vi "DashboardPush.vi"(5 "Joystick 0 Ref":T1, 7 "Joystick 1 Ref":T1) -> ()   [LabVIEW 2018]
uses:
  <vilib>/Rock Robotics/WPI/Joystick/WPI_JoystickDevRef.ctl
  <vilib>/Rock Robotics/WPI/Joystick/WPI_JoystickDeviceEnum.ctl
  1cd4df9d-07b4-47b1-9361-2cbb9b342794.vi
  3ad63815-9e92-4927-9537-e4f1665bbc86.vi
  3818bb57-508c-4caa-99a3-3627e757767c.vi
  6295dfb8-7bb5-4d21-8815-7d68ced149fe.vi
  69aab131-d86d-4f55-ad43-4766d5f58e80.vi
  c3e94fa6-8c65-408c-b4b8-dd7b71f991a8.vi
  26d44c84-0892-4d1c-ad1a-86279a09e0cc.vi
  6918a5f6-b485-4e67-ab72-405280ef4693.vi
  11adc3a0-d4d2-454d-8758-117694ddcb4c.vi
  1a812ba0-d878-476d-99f2-b93886c55b51.vi
  4ab55bdd-9685-40f0-9085-ecc7bf01abd7.vi
  133b72f1-f6b5-40a0-849f-8c3469abb341.vi
  418ca814-9bf7-4181-a5ae-ea4e15d15a62.vi
  5b9a1c80-d2af-4722-947b-ad6779bb500a.vi
  bbae46cd-89b0-4a78-83b4-a5d1ddadd6d9.vi
  6394f793-1348-457d-85f4-7648f9013d39.vi
  47d326fc-03e5-451f-ae34-c9ea74063880.vi
  a9e42ba8-a108-4121-8da4-7ed463bc445a.vi
  e7382db6-2398-4bf7-9509-2739849d011a.vi
  fb3d1e40-1309-4105-9d60-3501161224b8.vi
  edb44874-fd78-454c-9bff-6d2a69ee6fec.vi
  dfb785ac-7a80-4692-ab1e-e9791fae54f3.vi
  5b13cb5e-6146-47d8-ae09-8b12801406e1.vi
  221b1552-0cc4-4389-bc13-d572fc4176ac.vi
  30f734cc-7591-4d07-939c-c5b43ee5df0c.vi
  d7311573-fb90-4913-8cda-848d1d3ce53b.vi
  7ba6df12-c395-4848-b3a1-04dcd1203c1b.vi
  6301e614-6b7f-47cf-b382-4b27c7e33111.vi
  d83519f1-9582-40c6-a23b-344b6b305b5b.vi
  6aad11fd-ae03-4511-b650-1fa0753debfc.vi
  3bc1cfba-3c18-4848-9658-0328ea52b25d.vi
  ee07aba5-9db9-42ab-a6d0-ff6a71bb383e.vi
  31b97e73-c245-4c28-83b2-b8b7bc5cac65.vi
  8687fe65-8d2d-4f02-ae89-6e8600396bf0.vi
  359c22e3-9c88-41c1-8194-a7f6db251ab3.vi
  9a35cad7-8924-4936-b892-f51ff88f3087.vi
  77a43352-c56d-4a82-a601-0e029bfbecdd.vi
  6c32de76-4603-4c98-9548-18c068db77e4.vi
  fb2c5630-2057-4e14-823f-31378c39dbf8.vi
  d6cbd67f-9b17-42bf-843e-f5ce2d93bab6.vi
  9a319e29-0bce-4b5a-a8ba-81b1ec785933.vi
  c84b3921-0e7b-4db5-8b5b-9ca439e6cec8.vi
  80ca6acc-a426-4631-8635-04e987b8dcbd.vi
  32f607b5-8f1a-4da3-a9f3-63ceddb82894.vi
  SensorReadings.vi
  RobotStates.vi
  Inputs_DriverStation.vi
  <vilib>/Rock Robotics/Network Tables/NT Write Number.vi
  <vilib>/Rock Robotics/Network Tables/NT Write Boolean.vi
  Robot Global Data.vi
  <vilib>/Rock Robotics/Network Tables/NT Write String.vi
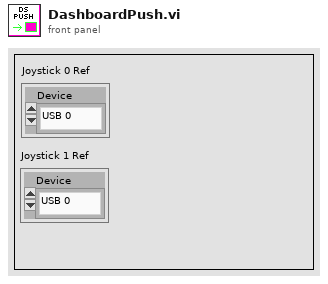
[diagram p1: front panel]
types:
  T1 = typedef "WPI_JoystickDevRef.ctl" = cluster{"Device":T2}
  T2 = typedef "WPI_JoystickDeviceEnum.ctl" = enum16{"USB 0", "USB 1", "USB 2", "USB 3", "USB 4", "USB 5"}
  T3 = cluster{"[0]":bool, "[1]":bool, "[2]":bool, "[3]":bool, "[4]":bool, "[5]":bool, "[6]":bool, "[7]":bool, "[8]":bool, "[9]":bool, "[10]":bool, "[11]":bool, "[12]":bool, "[13]":bool}
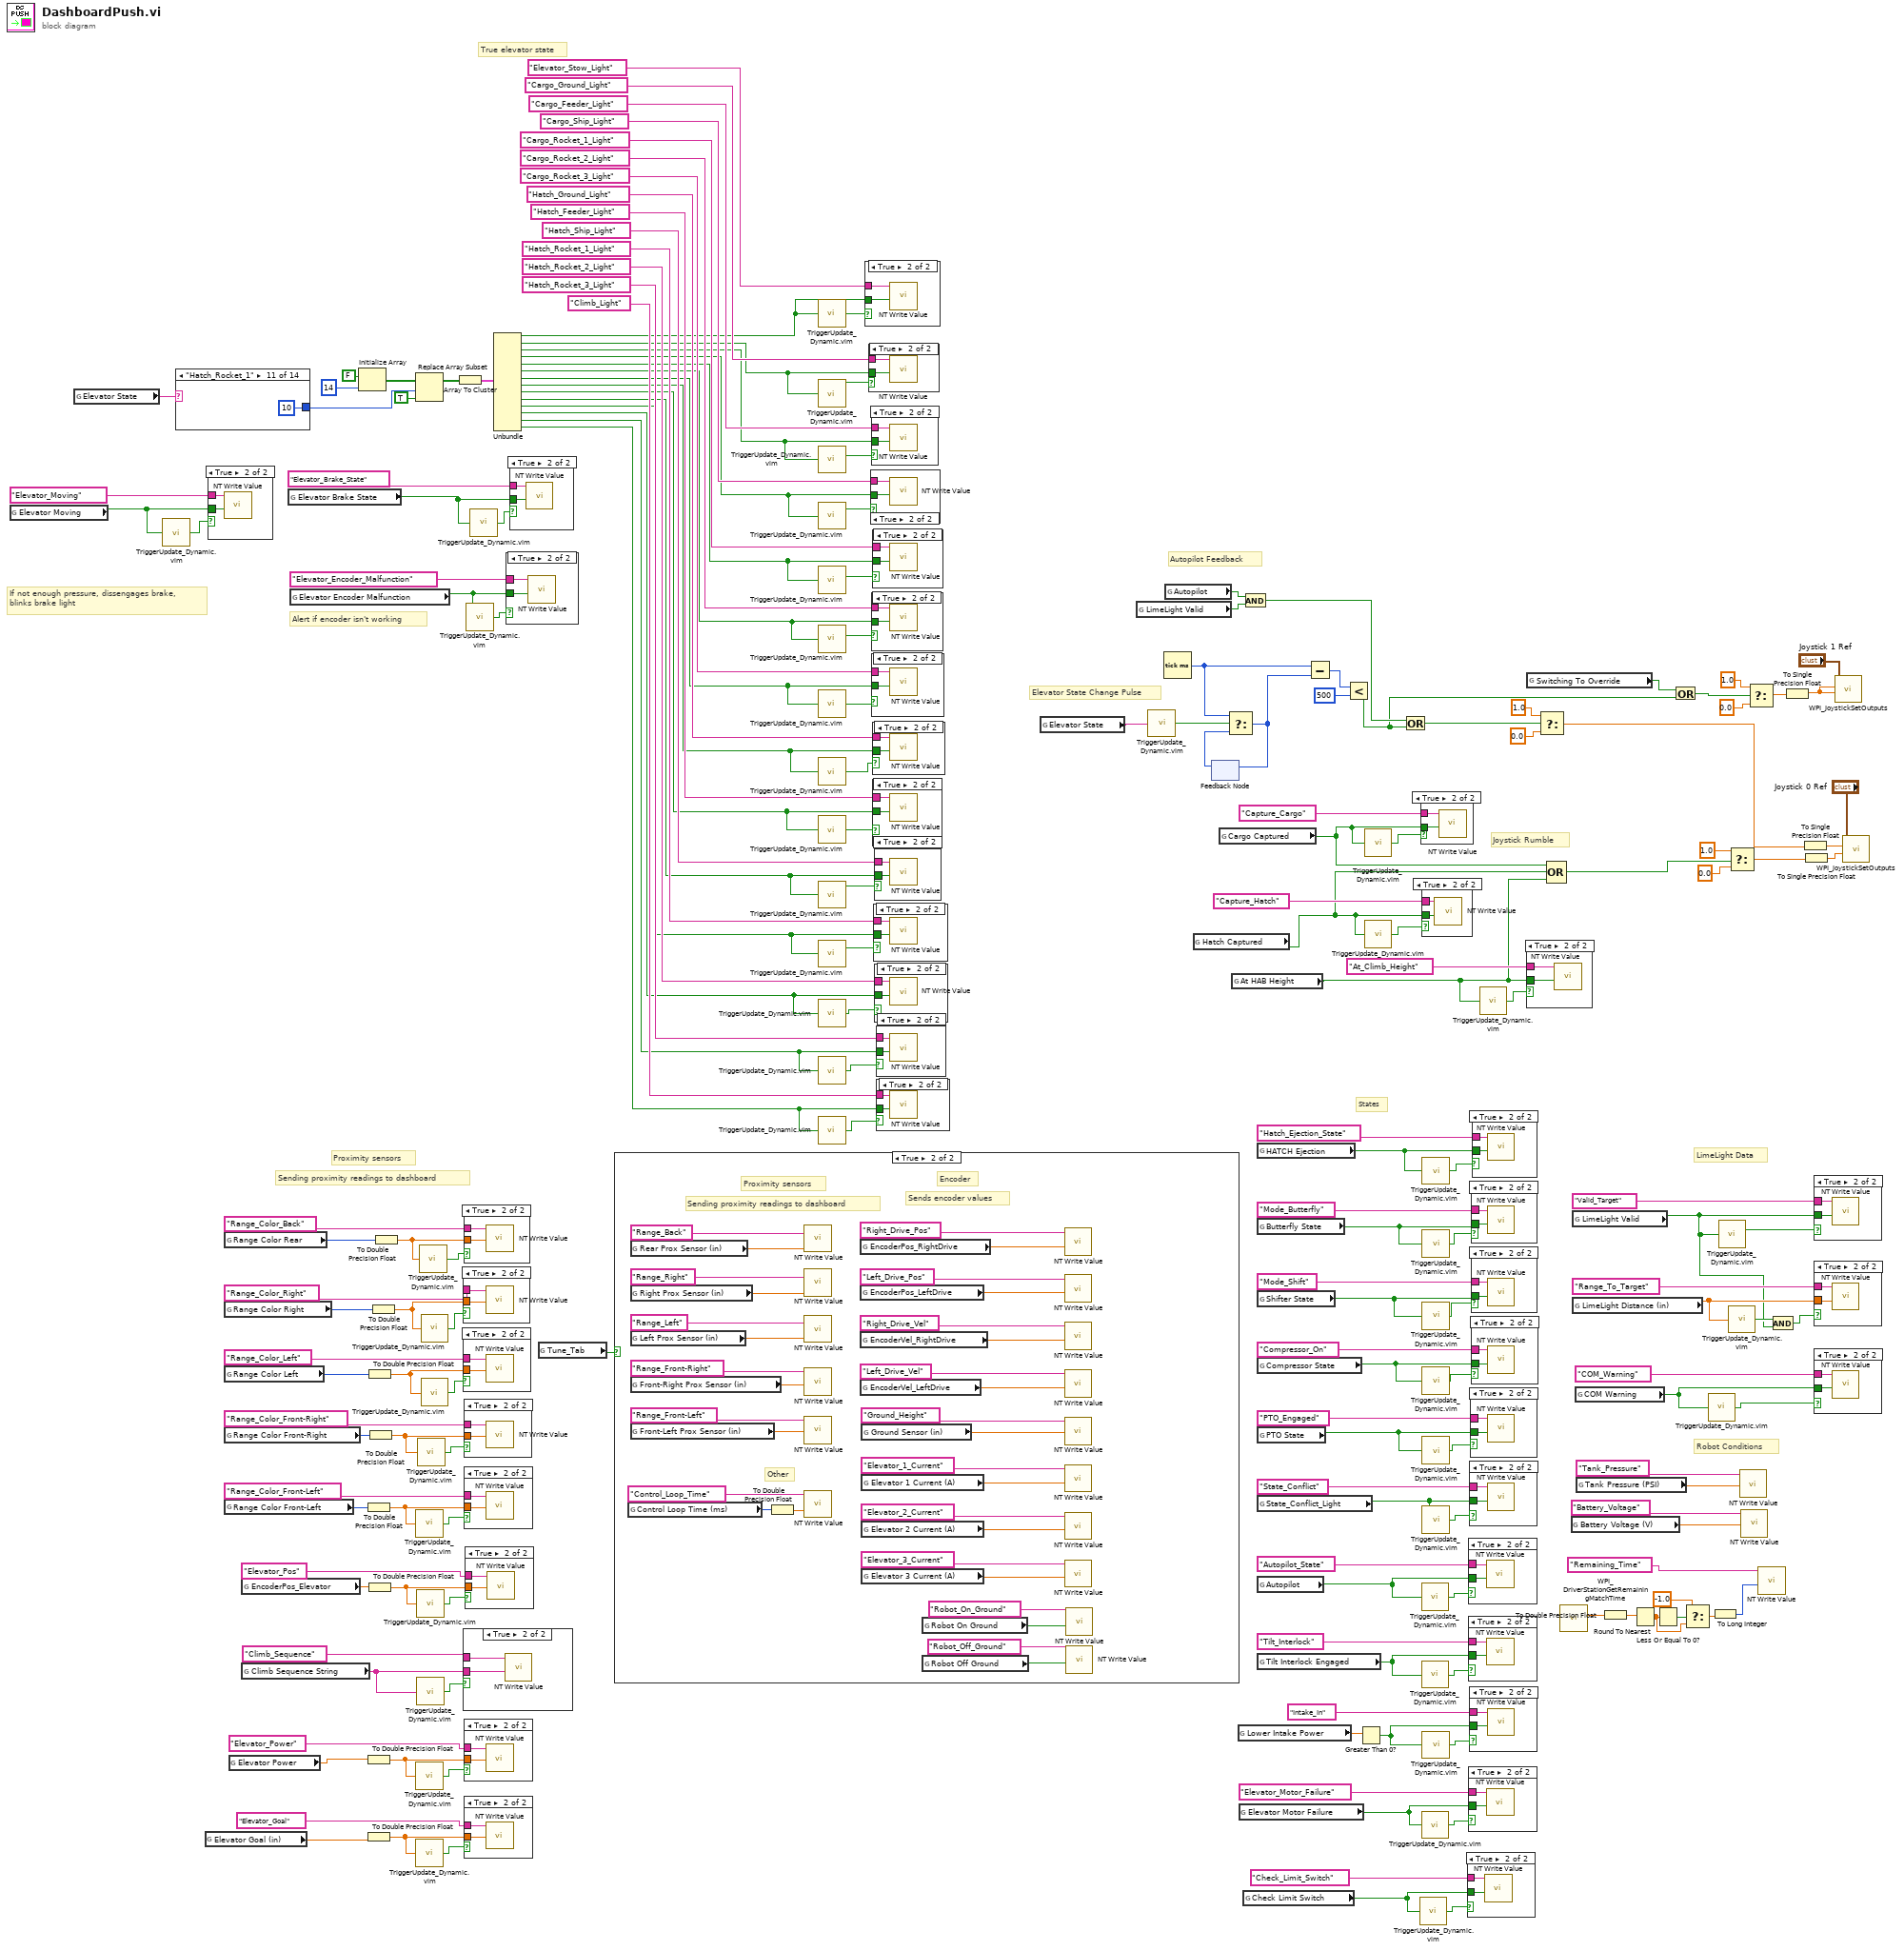
[diagram p0: block diagram]
diagram:
  # "Robot Conditions"
  # "States"
  # "Elevator State Change Pulse"
  # "LimeLight Data"
  # "Autopilot Feedback"
  # "Sending proximity readings to dashboard"
  # "Alert if encoder isn't working"
  # "If not enough pressure, dissengages brake,\nblinks brake light"
  # "Joystick Rumble"
  # "Proximity sensors"
  # "True elevator state"
  n1 = global read "RobotStates.vi" "Elevator Moving"() -> (w50:bool)
  n2 = global read "RobotStates.vi" "Elevator State"() -> (w156:string)
  n3 = call "TriggerUpdate_Dynamic.vim"("Trigger"=w50) -> ("Update"=w49:bool)
  n4 = case shown="\"Hatch_Rocket_1\"" w156 {
    tunnel: [0 1 2 3 4 5 6 7 8 9 10 11 12 13] -> w155
    frame "Elevator_Stow", Default {
    }
    frame "Cargo_Ground" {
    }
    frame "Cargo_Feeder" {
    }
    frame "Cargo_Ship" {
    }
    frame "Cargo_Rocket_1" {
    }
    frame "Cargo_Rocket_2" {
    }
    frame "Cargo_Rocket_3" {
    }
    frame "Hatch_Ground" {
    }
    frame "Hatch_Feeder" {
    }
    frame "Hatch_Ship" {
    }
    frame "Hatch_Rocket_1" {
    }
    frame "Hatch_Rocket_2" {
    }
    frame "Hatch_Rocket_3" {
    }
    frame "Climb" {
    }
  }
  n5 = global read "RobotStates.vi" "Elevator Goal (in)"() -> (w7:dbl)
  n6 = case shown="True" w49 {
    tunnel: "Elevator_Moving" ("Name") -> [_ w205]
    tunnel: w50 -> [_ w204]
    frame False {
    }
    frame True {
      n7 = call-poly <vilib>:"NT Write Value.vi"("Boolean"=w204, "Name"=w205) -> ()  [unwired: 9 in, 1 out]
    }
  }
  n8 = global read "SensorReadings.vi" "Range Color Rear"() -> (w182:u32)
  n9 = global read "SensorReadings.vi" "Range Color Right"() -> (w180:u32)
  n10 = global read "SensorReadings.vi" "Range Color Left"() -> (w178:u32)
  n11 = global read "SensorReadings.vi" "Range Color Front-Right"() -> (w176:u32)
  n12 = global read "SensorReadings.vi" "Range Color Front-Left"() -> (w151:u32)
  n13 = global read "RobotStates.vi" "Elevator Power"() -> (w11:dbl)
  n14 = global read "SensorReadings.vi" "EncoderPos_Elevator"() -> (w30:dbl)
  n15 = global read "RobotStates.vi" "Climb Sequence String"() -> (w27:string)
  n16 = global read "RobotStates.vi" "Elevator Brake State"() -> (w91:bool)
  n17 = global read "SensorReadings.vi" "Elevator Encoder Malfunction"() -> (w45:bool)
  n18 = Initialize Array(FALSE, 14 ("dimension size")) -> (w161:bool[])
  n19 = To Double Precision Float(number=w151) -> (double precision float=w95:dbl)
  n20 = To Double Precision Float(number=w11) -> (double precision float=w14:dbl)
  n21 = To Double Precision Float(number=w7) -> (double precision float=w10:dbl)
  n22 = To Double Precision Float(number=w178) -> (double precision float=w99:dbl)
  n23 = To Double Precision Float(number=w30) -> (double precision float=w33:dbl)
  n24 = To Double Precision Float(number=w176) -> (double precision float=w97:dbl)
  n25 = To Double Precision Float(number=w180) -> (double precision float=w101:dbl)
  n26 = To Double Precision Float(number=w182) -> (double precision float=w103:dbl)
  n27 = Replace Array Subset(array=w161, new element=TRUE ("new element/subarray"), index=w155) -> (w159:bool[])
  n28 = call "TriggerUpdate_Dynamic.vim"("Trigger"=w95) -> ("Update"=w94:bool)
  n29 = call "TriggerUpdate_Dynamic.vim"("Trigger"=w14) -> ("Update"=w13:bool)
  n30 = call "TriggerUpdate_Dynamic.vim"("Trigger"=w10) -> ("Update"=w9:bool)
  n31 = call "TriggerUpdate_Dynamic.vim"("Trigger"=w33) -> ("Update"=w32:bool)
  n32 = call "TriggerUpdate_Dynamic.vim"("Trigger"=w27) -> ("Update"=w29:bool)
  n33 = call "TriggerUpdate_Dynamic.vim"("Trigger"=w97) -> ("Update"=w96:bool)
  n34 = call "TriggerUpdate_Dynamic.vim"("Trigger"=w103) -> ("Update"=w102:bool)
  n35 = call "TriggerUpdate_Dynamic.vim"("Trigger"=w101) -> ("Update"=w100:bool)
  n36 = call "TriggerUpdate_Dynamic.vim"("Trigger"=w99) -> ("Update"=w98:bool)
  n37 = Array To Cluster(array=w159) -> (cluster=w158:T3)
  n38 = case shown="True" w100 {
    tunnel: "Range_Color_Right" ("refnum name") -> [_ w207]
    tunnel: w101 -> [_ w206]
    frame False {
    }
    frame True {
      n39 = call-poly <vilib>:"NT Write Value.vi"("Numeric"=w206, "Name"=w207) -> ()  [unwired: 9 in, 1 out]
    }
  }
  n40 = case shown="True" w98 {
    tunnel: "Range_Color_Left" ("refnum name") -> [_ w209]
    tunnel: w99 -> [_ w208]
    frame False {
    }
    frame True {
      n41 = call-poly <vilib>:"NT Write Value.vi"("Numeric"=w208, "Name"=w209) -> ()  [unwired: 9 in, 1 out]
    }
  }
  n42 = case shown="True" w29 {
    tunnel: "Climb_Sequence" ("Name") -> [_ w211]
    tunnel: w27 -> [_ w210]
    frame False {
    }
    frame True {
      n43 = call-poly <vilib>:"NT Write Value.vi"("String"=w210, "Name"=w211) -> ()  [unwired: 9 in, 1 out]
    }
  }
  n44 = case shown="True" w102 {
    tunnel: "Range_Color_Back" ("refnum name") -> [_ w213]
    tunnel: w103 -> [_ w212]
    frame False {
    }
    frame True {
      n45 = call-poly <vilib>:"NT Write Value.vi"("Numeric"=w212, "Name"=w213) -> ()  [unwired: 9 in, 1 out]
    }
  }
  n46 = case shown="True" w96 {
    tunnel: "Range_Color_Front-Right" ("refnum name") -> [_ w215]
    tunnel: w97 -> [_ w214]
    frame False {
    }
    frame True {
      n47 = call-poly <vilib>:"NT Write Value.vi"("Numeric"=w214, "Name"=w215) -> ()  [unwired: 9 in, 1 out]
    }
  }
  n48 = case shown="True" w94 {
    tunnel: w95 -> [_ w217]
    tunnel: "Range_Color_Front-Left" ("refnum name") -> [_ w216]
    frame False {
    }
    frame True {
      n49 = call-poly <vilib>:"NT Write Value.vi"("Numeric"=w217, "Name"=w216) -> ()  [unwired: 9 in, 1 out]
    }
  }
  n50 = case shown="True" w13 {
    tunnel: w14 -> [_ w219]
    tunnel: "Elevator_Power" ("Name") -> [_ w218]
    frame False {
    }
    frame True {
      n51 = call-poly <vilib>:"NT Write Value.vi"("Numeric"=w219, "Name"=w218) -> ()  [unwired: 9 in, 1 out]
    }
  }
  n52 = case shown="True" w9 {
    tunnel: w10 -> [_ w221]
    tunnel: "Elevator_Goal" ("Name") -> [_ w220]
    frame False {
    }
    frame True {
      n53 = call-poly <vilib>:"NT Write Value.vi"("Numeric"=w221, "Name"=w220) -> ()  [unwired: 9 in, 1 out]
    }
  }
  n54 = case shown="True" w32 {
    tunnel: w33 -> [_ w223]
    tunnel: "Elevator_Pos" ("Name") -> [_ w222]
    frame False {
    }
    frame True {
      n55 = call-poly <vilib>:"NT Write Value.vi"("Numeric"=w223, "Name"=w222) -> ()  [unwired: 9 in, 1 out]
    }
  }
  n56 = call "TriggerUpdate_Dynamic.vim"("Trigger"=w45) -> ("Update"=w92:bool)
  n57 = call "TriggerUpdate_Dynamic.vim"("Trigger"=w91) -> ("Update"=w90:bool)
  n58 = Unbundle(w158) -> ("[0]"=w146:bool, "[1]"=w144:bool, "[2]"=w142:bool, "[3]"=w140:bool, "[4]"=w138:bool, "[5]"=w136:bool, "[6]"=w134:bool, "[7]"=w132:bool, "[8]"=w130:bool, "[9]"=w128:bool, "[10]"=w126:bool, "[11]"=w124:bool, "[12]"=w122:bool, "[13]"=w120:bool)
  n59 = case shown="True" w92 {
    tunnel: "Elevator_Encoder_Malfunction" ("Name") -> [_ w225]
    tunnel: w45 -> [_ w224]
    frame False {
    }
    frame True {
      n60 = call-poly <vilib>:"NT Write Value.vi"("Boolean"=w224, "Name"=w225) -> ()  [unwired: 9 in, 1 out]
    }
  }
  n61 = case shown="True" w90 {
    tunnel: "Elevator_Brake_State" ("Name") -> [_ w227]
    tunnel: w91 -> [_ w226]
    frame False {
    }
    frame True {
      n62 = call-poly <vilib>:"NT Write Value.vi"("Boolean"=w226, "Name"=w227) -> ()  [unwired: 9 in, 1 out]
    }
  }
  n63 = global read "Inputs_DriverStation.vi" "Tune_Tab"() -> (w93:bool)
  n64 = case shown="True" w93 {
    frame False {
    }
    frame True {
      # "Sending proximity readings to dashboard"
      # "Proximity sensors"
      # "Sends encoder values"
      # "Other"
      # "Encoder"
      n65 = global read "SensorReadings.vi" "Control Loop Time (ms)"() -> (w241:u32)
      n66 = global read "SensorReadings.vi" "Rear Prox Sensor (in)"() -> (w259:dbl)
      n67 = global read "SensorReadings.vi" "Right Prox Sensor (in)"() -> (w257:dbl)
      n68 = global read "SensorReadings.vi" "Left Prox Sensor (in)"() -> (w255:dbl)
      n69 = global read "SensorReadings.vi" "Front-Right Prox Sensor (in)"() -> (w253:dbl)
      n70 = global read "SensorReadings.vi" "Front-Left Prox Sensor (in)"() -> (w243:dbl)
      n71 = To Double Precision Float(number=w241) -> (double precision float=w240:dbl)
      n72 = call-poly <vilib>:"NT Write Value.vi"("Numeric"=w259, "Name"="Range_Back") -> ()  [unwired: 9 in, 1 out]
      n73 = call-poly <vilib>:"NT Write Value.vi"("Numeric"=w257, "Name"="Range_Right") -> ()  [unwired: 9 in, 1 out]
      n74 = call-poly <vilib>:"NT Write Value.vi"("Numeric"=w255, "Name"="Range_Left") -> ()  [unwired: 9 in, 1 out]
      n75 = call-poly <vilib>:"NT Write Value.vi"("Numeric"=w253, "Name"="Range_Front-Right") -> ()  [unwired: 9 in, 1 out]
      n76 = call-poly <vilib>:"NT Write Value.vi"("Numeric"=w243, "Name"="Range_Front-Left") -> ()  [unwired: 9 in, 1 out]
      n77 = call-poly <vilib>:"NT Write Value.vi"("Numeric"=w240, "Name"="Control_Loop_Time") -> ()  [unwired: 9 in, 1 out]
      n78 = global read "SensorReadings.vi" "EncoderPos_RightDrive"() -> (w252:dbl)
      n79 = global read "SensorReadings.vi" "EncoderPos_LeftDrive"() -> (w250:dbl)
      n80 = global read "SensorReadings.vi" "EncoderVel_RightDrive"() -> (w248:dbl)
      n81 = global read "SensorReadings.vi" "EncoderVel_LeftDrive"() -> (w246:dbl)
      n82 = global read "SensorReadings.vi" "Ground Sensor (in)"() -> (w238:dbl)
      n83 = global read "SensorReadings.vi" "Elevator 1 Current (A)"() -> (w236:dbl)
      n84 = global read "SensorReadings.vi" "Elevator 2 Current (A)"() -> (w234:dbl)
      n85 = global read "SensorReadings.vi" "Elevator 3 Current (A)"() -> (w232:dbl)
      n86 = global read "SensorReadings.vi" "Robot On Ground"() -> (w230:bool)
      n87 = global read "SensorReadings.vi" "Robot Off Ground"() -> (w231:bool)
      n88 = call-poly <vilib>:"NT Write Value.vi"("Numeric"=w252, "Name"="Right_Drive_Pos") -> ()  [unwired: 9 in, 1 out]
      n89 = call-poly <vilib>:"NT Write Value.vi"("Numeric"=w250, "Name"="Left_Drive_Pos") -> ()  [unwired: 9 in, 1 out]
      n90 = call-poly <vilib>:"NT Write Value.vi"("Numeric"=w248, "Name"="Right_Drive_Vel") -> ()  [unwired: 9 in, 1 out]
      n91 = call-poly <vilib>:"NT Write Value.vi"("Numeric"=w246, "Name"="Left_Drive_Vel") -> ()  [unwired: 9 in, 1 out]
      n92 = call-poly <vilib>:"NT Write Value.vi"("Numeric"=w238, "Name"="Ground_Height") -> ()  [unwired: 9 in, 1 out]
      n93 = call-poly <vilib>:"NT Write Value.vi"("Numeric"=w236, "Name"="Elevator_1_Current") -> ()  [unwired: 9 in, 1 out]
      n94 = call-poly <vilib>:"NT Write Value.vi"("Numeric"=w234, "Name"="Elevator_2_Current") -> ()  [unwired: 9 in, 1 out]
      n95 = call-poly <vilib>:"NT Write Value.vi"("Numeric"=w232, "Name"="Elevator_3_Current") -> ()  [unwired: 9 in, 1 out]
      n96 = call-poly <vilib>:"NT Write Value.vi"("Boolean"=w230, "Name"="Robot_On_Ground") -> ()  [unwired: 9 in, 1 out]
      n97 = call-poly <vilib>:"NT Write Value.vi"("Boolean"=w231, "Name"="Robot_Off_Ground") -> ()  [unwired: 9 in, 1 out]
    }
  }
  n98 = call "TriggerUpdate_Dynamic.vim"("Trigger"=w146) -> ("Update"=w145:bool)
  n99 = call "TriggerUpdate_Dynamic.vim"("Trigger"=w144) -> ("Update"=w143:bool)
  n100 = call "TriggerUpdate_Dynamic.vim"("Trigger"=w142) -> ("Update"=w141:bool)
  n101 = call "TriggerUpdate_Dynamic.vim"("Trigger"=w140) -> ("Update"=w139:bool)
  n102 = call "TriggerUpdate_Dynamic.vim"("Trigger"=w138) -> ("Update"=w137:bool)
  n103 = call "TriggerUpdate_Dynamic.vim"("Trigger"=w136) -> ("Update"=w135:bool)
  n104 = call "TriggerUpdate_Dynamic.vim"("Trigger"=w134) -> ("Update"=w133:bool)
  n105 = call "TriggerUpdate_Dynamic.vim"("Trigger"=w132) -> ("Update"=w131:bool)
  n106 = call "TriggerUpdate_Dynamic.vim"("Trigger"=w130) -> ("Update"=w129:bool)
  n107 = call "TriggerUpdate_Dynamic.vim"("Trigger"=w128) -> ("Update"=w127:bool)
  n108 = call "TriggerUpdate_Dynamic.vim"("Trigger"=w126) -> ("Update"=w125:bool)
  n109 = call "TriggerUpdate_Dynamic.vim"("Trigger"=w124) -> ("Update"=w123:bool)
  n110 = call "TriggerUpdate_Dynamic.vim"("Trigger"=w122) -> ("Update"=w121:bool)
  n111 = call "TriggerUpdate_Dynamic.vim"("Trigger"=w120) -> ("Update"=w119:bool)
  n112 = case shown="True" w145 {
    tunnel: "Elevator_Stow_Light" ("refnum name") -> [_ w262]
    tunnel: w146 -> [_ w261]
    frame False {
    }
    frame True {
      n113 = call-poly <vilib>:"NT Write Value.vi"("Boolean"=w261, "Name"=w262) -> ()  [unwired: 9 in, 1 out]
    }
  }
  n114 = case shown="True" w143 {
    tunnel: "Cargo_Ground_Light" ("refnum name") -> [_ w264]
    tunnel: w144 -> [_ w263]
    frame False {
    }
    frame True {
      n115 = call-poly <vilib>:"NT Write Value.vi"("Boolean"=w263, "Name"=w264) -> ()  [unwired: 9 in, 1 out]
    }
  }
  n116 = case shown="True" w139 {
    tunnel: "Cargo_Ship_Light" ("refnum name") -> [_ w266]
    tunnel: w140 -> [_ w265]
    frame False {
    }
    frame True {
      n117 = call-poly <vilib>:"NT Write Value.vi"("Boolean"=w265, "Name"=w266) -> ()  [unwired: 9 in, 1 out]
    }
  }
  n118 = case shown="True" w141 {
    tunnel: "Cargo_Feeder_Light" ("refnum name") -> [_ w268]
    tunnel: w142 -> [_ w267]
    frame False {
    }
    frame True {
      n119 = call-poly <vilib>:"NT Write Value.vi"("Boolean"=w267, "Name"=w268) -> ()  [unwired: 9 in, 1 out]
    }
  }
  n120 = case shown="True" w135 {
    tunnel: "Cargo_Rocket_2_Light" ("refnum name") -> [_ w270]
    tunnel: w136 -> [_ w269]
    frame False {
    }
    frame True {
      n121 = call-poly <vilib>:"NT Write Value.vi"("Boolean"=w269, "Name"=w270) -> ()  [unwired: 9 in, 1 out]
    }
  }
  n122 = case shown="True" w133 {
    tunnel: "Cargo_Rocket_3_Light" ("refnum name") -> [_ w272]
    tunnel: w134 -> [_ w271]
    frame False {
    }
    frame True {
      n123 = call-poly <vilib>:"NT Write Value.vi"("Boolean"=w271, "Name"=w272) -> ()  [unwired: 9 in, 1 out]
    }
  }
  n124 = case shown="True" w137 {
    tunnel: "Cargo_Rocket_1_Light" ("refnum name") -> [_ w274]
    tunnel: w138 -> [_ w273]
    frame False {
    }
    frame True {
      n125 = call-poly <vilib>:"NT Write Value.vi"("Boolean"=w273, "Name"=w274) -> ()  [unwired: 9 in, 1 out]
    }
  }
  n126 = case shown="True" w131 {
    tunnel: "Hatch_Ground_Light" ("refnum name") -> [_ w276]
    tunnel: w132 -> [_ w275]
    frame False {
    }
    frame True {
      n127 = call-poly <vilib>:"NT Write Value.vi"("Boolean"=w275, "Name"=w276) -> ()  [unwired: 9 in, 1 out]
    }
  }
  n128 = case shown="True" w129 {
    tunnel: "Hatch_Feeder_Light" ("refnum name") -> [_ w278]
    tunnel: w130 -> [_ w277]
    frame False {
    }
    frame True {
      n129 = call-poly <vilib>:"NT Write Value.vi"("Boolean"=w277, "Name"=w278) -> ()  [unwired: 9 in, 1 out]
    }
  }
  n130 = case shown="True" w125 {
    tunnel: "Hatch_Rocket_1_Light" ("refnum name") -> [_ w280]
    tunnel: w126 -> [_ w279]
    frame False {
    }
    frame True {
      n131 = call-poly <vilib>:"NT Write Value.vi"("Boolean"=w279, "Name"=w280) -> ()  [unwired: 9 in, 1 out]
    }
  }
  n132 = case shown="True" w127 {
    tunnel: "Hatch_Ship_Light" ("refnum name") -> [_ w282]
    tunnel: w128 -> [_ w281]
    frame False {
    }
    frame True {
      n133 = call-poly <vilib>:"NT Write Value.vi"("Boolean"=w281, "Name"=w282) -> ()  [unwired: 9 in, 1 out]
    }
  }
  n134 = case shown="True" w123 {
    tunnel: "Hatch_Rocket_2_Light" ("refnum name") -> [_ w284]
    tunnel: w124 -> [_ w283]
    frame False {
    }
    frame True {
      n135 = call-poly <vilib>:"NT Write Value.vi"("Boolean"=w283, "Name"=w284) -> ()  [unwired: 9 in, 1 out]
    }
  }
  n136 = case shown="True" w121 {
    tunnel: "Hatch_Rocket_3_Light" ("refnum name") -> [_ w286]
    tunnel: w122 -> [_ w285]
    frame False {
    }
    frame True {
      n137 = call-poly <vilib>:"NT Write Value.vi"("Boolean"=w285, "Name"=w286) -> ()  [unwired: 9 in, 1 out]
    }
  }
  n138 = case shown="True" w119 {
    tunnel: "Climb_Light" ("refnum name") -> [_ w288]
    tunnel: w120 -> [_ w287]
    frame False {
    }
    frame True {
      n139 = call-poly <vilib>:"NT Write Value.vi"("Boolean"=w287, "Name"=w288) -> ()  [unwired: 9 in, 1 out]
    }
  }
  n140 = global read "RobotStates.vi" "Elevator State"() -> (w65:string)
  n141 = global read "SensorReadings.vi" "LimeLight Valid"() -> (w88:bool)
  n142 = call "TriggerUpdate_Dynamic.vim"("Trigger"=w65) -> ("Update"=w57:bool)
  n143 = Tick Count (ms)() -> (millisecond timer value=w61:u32)
  n144 = global read "RobotStates.vi" "Autopilot"() -> (w89:bool)
  n145 = global read "SensorReadings.vi" "Hatch Captured"() -> (w66:bool)
  n146 = feedback #1() -> (w62:u32)  [unwired: 1 in]
  n147 = global read "SensorReadings.vi" "Cargo Captured"() -> (w117:bool)
  n148 = Select(t=w61, s=w57, f=w62) -> (s? t:f=w60:u32)
  n149 = feedback-in #1(w60) -> ()
  n150 = global read "SensorReadings.vi" "At HAB Height"() -> (w34:bool)
  n151 = global read "RobotStates.vi" "Lower Intake Power"() -> (w24:dbl)
  n152 = global read "RobotStates.vi" "Elevator Motor Failure"() -> (w4:bool)
  n153 = And(x=w89, y=w88) -> (x .and. y?=w64:bool)
  n154 = global read "RobotStates.vi" "Check Limit Switch"() -> (w1:bool)
  n155 = global read "RobotStates.vi" "HATCH Ejection"() -> (w115:bool)
  n156 = global read "RobotStates.vi" "Butterfly State"() -> (w113:bool)
  n157 = global read "RobotStates.vi" "Shifter State"() -> (w111:bool)
  n158 = global read "RobotStates.vi" "Compressor State"() -> (w109:bool)
  n159 = global read "RobotStates.vi" "PTO State"() -> (w107:bool)
  n160 = global read "RobotStates.vi" "State_Conflict_Light"() -> (w105:bool)
  n161 = global read "RobotStates.vi" "Autopilot"() -> (w77:bool)
  n162 = global read "RobotStates.vi" "Tilt Interlock Engaged"() -> (w41:bool)
  n163 = Subtract(x=w61, y=w60) -> (x-y=w59:u32)
  n164 = Less?(x=w59, y=u32 500) -> (x < y?=w39:bool)
  n165 = Greater Than 0?(x=w24) -> (x > 0?=w23:bool)
  n166 = call "TriggerUpdate_Dynamic.vim"("Trigger"=w117) -> ("Update"=w116:bool)
  n167 = call "TriggerUpdate_Dynamic.vim"("Trigger"=w66) -> ("Update"=w118:bool)
  n168 = Or(x=w64, y=w39) -> (x .or. y?=w63:bool)
  n169 = call "TriggerUpdate_Dynamic.vim"("Trigger"=w1) -> ("Update"=w2:bool)
  n170 = case shown="True" w116 {
    tunnel: "Capture_Cargo" ("Name") -> [_ w290]
    tunnel: w117 -> [_ w289]
    frame False {
    }
    frame True {
      n171 = call-poly <vilib>:"NT Write Value.vi"("Boolean"=w289, "Name"=w290) -> ()  [unwired: 9 in, 1 out]
    }
  }
  n172 = call "TriggerUpdate_Dynamic.vim"("Trigger"=w77) -> ("Update"=w76:bool)
  n173 = call "TriggerUpdate_Dynamic.vim"("Trigger"=w41) -> ("Update"=w40:bool)
  n174 = call "TriggerUpdate_Dynamic.vim"("Trigger"=w4) -> ("Update"=w5:bool)
  n175 = case shown="True" w118 {
    tunnel: "Capture_Hatch" ("Name") -> [_ w292]
    tunnel: w66 -> [_ w291]
    frame False {
    }
    frame True {
      n176 = call-poly <vilib>:"NT Write Value.vi"("Boolean"=w291, "Name"=w292) -> ()  [unwired: 9 in, 1 out]
    }
  }
  n177 = call "TriggerUpdate_Dynamic.vim"("Trigger"=w115) -> ("Update"=w114:bool)
  n178 = call "TriggerUpdate_Dynamic.vim"("Trigger"=w113) -> ("Update"=w112:bool)
  n179 = call "TriggerUpdate_Dynamic.vim"("Trigger"=w111) -> ("Update"=w110:bool)
  n180 = call "TriggerUpdate_Dynamic.vim"("Trigger"=w109) -> ("Update"=w108:bool)
  n181 = call "TriggerUpdate_Dynamic.vim"("Trigger"=w107) -> ("Update"=w106:bool)
  n182 = call "TriggerUpdate_Dynamic.vim"("Trigger"=w105) -> ("Update"=w104:bool)
  n183 = call "TriggerUpdate_Dynamic.vim"("Trigger"=w23) -> ("Update"=w25:bool)
  n184 = case shown="True" w2 {
    tunnel: w1 -> [_ w294]
    tunnel: "Check_Limit_Switch" ("Name") -> [_ w293]
    frame False {
    }
    frame True {
      n185 = call-poly <vilib>:"NT Write Value.vi"("Boolean"=w294, "Name"=w293) -> ()  [unwired: 9 in, 1 out]
    }
  }
  n186 = case shown="True" w76 {
    tunnel: w77 -> [_ w296]
    tunnel: "Autopilot_State" ("Name") -> [_ w295]
    frame False {
    }
    frame True {
      n187 = call-poly <vilib>:"NT Write Value.vi"("Boolean"=w296, "Name"=w295) -> ()  [unwired: 9 in, 1 out]
    }
  }
  n188 = case shown="True" w40 {
    tunnel: w41 -> [_ w298]
    tunnel: "Tilt_Interlock" ("Name") -> [_ w297]
    frame False {
    }
    frame True {
      n189 = call-poly <vilib>:"NT Write Value.vi"("Boolean"=w298, "Name"=w297) -> ()  [unwired: 9 in, 1 out]
    }
  }
  n190 = case shown="True" w5 {
    tunnel: w4 -> [_ w300]
    tunnel: "Elevator_Motor_Failure" ("Name") -> [_ w299]
    frame False {
    }
    frame True {
      n191 = call-poly <vilib>:"NT Write Value.vi"("Boolean"=w300, "Name"=w299) -> ()  [unwired: 9 in, 1 out]
    }
  }
  n192 = case shown="True" w104 {
    tunnel: w105 -> [_ w302]
    tunnel: "State_Conflict" ("Name") -> [_ w301]
    frame False {
    }
    frame True {
      n193 = call-poly <vilib>:"NT Write Value.vi"("Boolean"=w302, "Name"=w301) -> ()  [unwired: 9 in, 1 out]
    }
  }
  n194 = case shown="True" w25 {
    tunnel: w23 -> [_ w304]
    tunnel: "Intake_In" ("Name") -> [_ w303]
    frame False {
    }
    frame True {
      n195 = call-poly <vilib>:"NT Write Value.vi"("Boolean"=w304, "Name"=w303) -> ()  [unwired: 9 in, 1 out]
    }
  }
  n196 = case shown="True" w106 {
    tunnel: "PTO_Engaged" ("Name") -> [_ w306]
    tunnel: w107 -> [_ w305]
    frame False {
    }
    frame True {
      n197 = call-poly <vilib>:"NT Write Value.vi"("Boolean"=w305, "Name"=w306) -> ()  [unwired: 9 in, 1 out]
    }
  }
  n198 = case shown="True" w112 {
    tunnel: "Mode_Butterfly" ("Name") -> [_ w308]
    tunnel: w113 -> [_ w307]
    frame False {
    }
    frame True {
      n199 = call-poly <vilib>:"NT Write Value.vi"("Boolean"=w307, "Name"=w308) -> ()  [unwired: 9 in, 1 out]
    }
  }
  n200 = case shown="True" w110 {
    tunnel: "Mode_Shift" ("Name") -> [_ w310]
    tunnel: w111 -> [_ w309]
    frame False {
    }
    frame True {
      n201 = call-poly <vilib>:"NT Write Value.vi"("Boolean"=w309, "Name"=w310) -> ()  [unwired: 9 in, 1 out]
    }
  }
  n202 = case shown="True" w108 {
    tunnel: "Compressor_On" ("Name") -> [_ w312]
    tunnel: w109 -> [_ w311]
    frame False {
    }
    frame True {
      n203 = call-poly <vilib>:"NT Write Value.vi"("Boolean"=w311, "Name"=w312) -> ()  [unwired: 9 in, 1 out]
    }
  }
  n204 = case shown="True" w114 {
    tunnel: "Hatch_Ejection_State" ("Name") -> [_ w314]
    tunnel: w115 -> [_ w313]
    frame False {
    }
    frame True {
      n205 = call-poly <vilib>:"NT Write Value.vi"("Boolean"=w313, "Name"=w314) -> ()  [unwired: 9 in, 1 out]
    }
  }
  n206 = call "TriggerUpdate_Dynamic.vim"("Trigger"=w34) -> ("Update"=w35:bool)
  n207 = global read "Inputs_DriverStation.vi" "Switching To Override"() -> (w37:bool)
  n208 = case shown="True" w35 {
    tunnel: "At_Climb_Height" ("Name") -> [_ w316]
    tunnel: w34 -> [_ w315]
    frame False {
    }
    frame True {
      n209 = call-poly <vilib>:"NT Write Value.vi"("Boolean"=w315, "Name"=w316) -> ()  [unwired: 9 in, 1 out]
    }
  }
  n210 = Select(t=1.0, s=w63, f=0.0) -> (s? t:f=w81:dbl)
  n211 = Compound Arithmetic op=OR(w117, w66, w34) -> (w79:bool)
  n212 = call <vilib>:"WPI_DriverStationGetRemainingMatchTime.vi"() -> ("Match Time(s)"=w21:sgl)  [unwired: 10 in, 1 out]
  n213 = global read "SensorReadings.vi" "Battery Voltage (V)"() -> (w44:dbl)
  n214 = global read "SensorReadings.vi" "LimeLight Valid"() -> (w69:bool)
  n215 = global read "SensorReadings.vi" "LimeLight Distance (in)"() -> (w72:dbl)
  n216 = global read "RobotStates.vi" "COM Warning"() -> (w47:bool)
  n217 = global read "SensorReadings.vi" "Tank Pressure (PSI)"() -> (w68:dbl)
  n218 = To Double Precision Float(number=w21) -> (double precision float=w20:dbl)
  n219 = Round To Nearest(number=w20) -> (nearest integer value=w18:dbl)
  n220 = Less Or Equal To 0?(x=w18) -> (x <= 0?=w19:bool)
  n221 = Or(x=w37, y=w39) -> (x .or. y?=w38:bool)
  n222 = Select(t=-1.0, s=w19, f=w18) -> (s? t:f=w17:dbl)
  n223 = call "TriggerUpdate_Dynamic.vim"("Trigger"=w47) -> ("Update"=w46:bool)
  n224 = To Long Integer(number=w17) -> (32bit integer=w16:i32)
  n225 = call "TriggerUpdate_Dynamic.vim"("Trigger"=w69) -> ("Update"=w74:bool)
  n226 = Select(t=1.0, s=w79, f=0.0) -> (s? t:f=w80:dbl)
  n227 = call "TriggerUpdate_Dynamic.vim"("Trigger"=w72) -> ("Update"=w71:bool)
  n228 = call-poly <vilib>:"NT Write Value.vi"("Numeric"=w68, "Name"="Tank_Pressure") -> ()  [unwired: 9 in, 1 out]
  n229 = call-poly <vilib>:"NT Write Value.vi"("Numeric"=w44, "Name"="Battery_Voltage") -> ()  [unwired: 9 in, 1 out]
  n230 = Select(t=1.0, s=w38, f=0.0) -> (s? t:f=w54:dbl)
  n231 = call-poly <vilib>:"NT Write Value.vi"("Numeric"=w16, "Name"="Remaining_Time") -> ()  [unwired: 9 in, 1 out]
  n232 = And(x=w71, y=w69) -> (x .and. y?=w70:bool)
  n233 = To Single Precision Float(number=w54) -> (single precision float=w52:sgl)
  n234 = To Single Precision Float(number=w81) -> (single precision float=w85:sgl)
  n235 = To Single Precision Float(number=w80) -> (single precision float=w82:sgl)
  n236 = case shown="True" w74 {
    tunnel: w69 -> [_ w318]
    tunnel: "Valid_Target" ("Name") -> [_ w317]
    frame False {
    }
    frame True {
      n237 = call-poly <vilib>:"NT Write Value.vi"("Boolean"=w318, "Name"=w317) -> ()  [unwired: 9 in, 1 out]
    }
  }
  n238 = case shown="True" w70 {
    tunnel: w72 -> [_ w320]
    tunnel: "Range_To_Target" ("Name") -> [_ w319]
    frame False {
    }
    frame True {
      n239 = call-poly <vilib>:"NT Write Value.vi"("Numeric"=w320, "Name"=w319) -> ()  [unwired: 9 in, 1 out]
    }
  }
  n240 = case shown="True" w46 {
    tunnel: w47 -> [_ w322]
    tunnel: "COM_Warning" ("Name") -> [_ w321]
    frame False {
    }
    frame True {
      n241 = call-poly <vilib>:"NT Write Value.vi"("Boolean"=w322, "Name"=w321) -> ()  [unwired: 9 in, 1 out]
    }
  }
  n242 = call <vilib>:"WPI_JoystickSetOutputs.vi"("Right Rumble"=w52, "Left Rumble"=w52, "JoystickDevRef"="Joystick 1 Ref") -> ()  [unwired: 7 in, 2 out]
  n243 = call <vilib>:"WPI_JoystickSetOutputs.vi"("Right Rumble"=w82, "Left Rumble"=w85, "JoystickDevRef"="Joystick 0 Ref") -> ()  [unwired: 7 in, 2 out]
